vi "GEA2 Script_Parser.vi"(0 "Script path":path, 5 "Default wait time (sec)":dbl=0.25 format="%#_13g", 7 "Default continue if failed?":bool, 11 "Error In":errorcluster) -> (4 "Script Output":T1[](array[typedef]), 6 "GEA2 Script":string, 15 "Error Out":errorcluster)   [LabVIEW 2014]
uses:
  typedefs/Script Output.ctl
  typedefs/Command Type.ctl
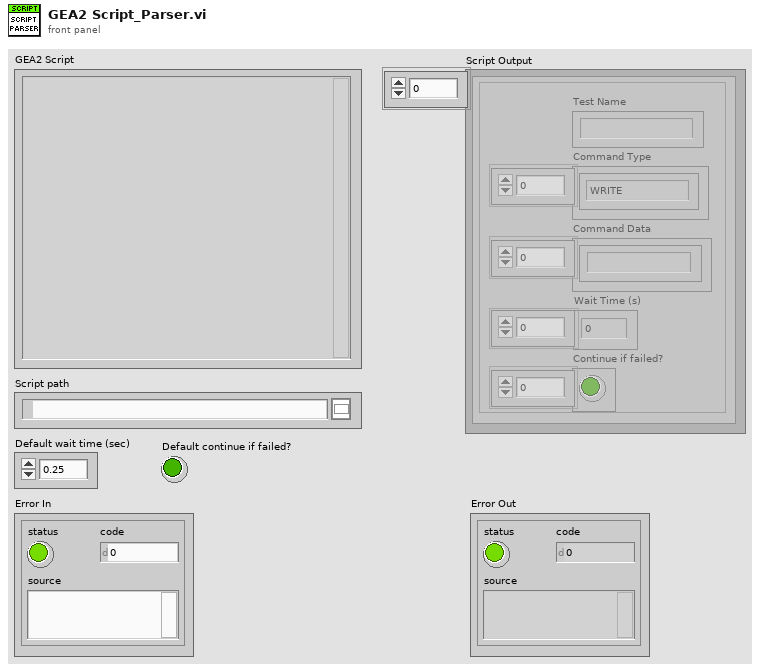
[diagram p1: front panel]
types:
  T1 = typedef "Script Output.ctl" = cluster{"Command Data":string[], "Command Type":T2[], "Test Name":string, "Wait Time (s)":dbl[], "Continue if failed?":bool[]}
  T2 = typedef "Command Type.ctl" = enum16{"WRITE", "READ", "ERDWRITE", "ERDREAD"}
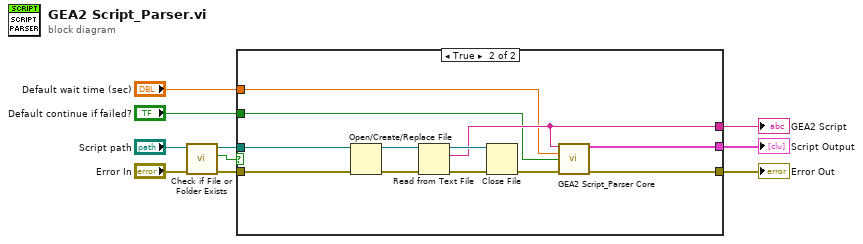
[diagram p0: block diagram]
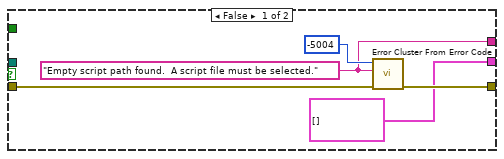
[diagram p2: hidden frame]
diagram:
  n1 = call <vilib>:"Check if File or Folder Exists.vi"("error in (no error)"="Error In", "path"="Script path") -> ("error out"=w7:errorcluster, "file or folder exists?"=w4:bool, "dup path"=w6:path)  [unwired: 7 in]
  n2 = case shown="True" w4 {
    tunnel: w7 -> [w14 w27]
    tunnel: [w15 w19] -> w10
    tunnel: "Default wait time (sec)" -> [_ w18]
    tunnel: w6 -> [_ w22]
    tunnel: [w12 w20] -> w3
    tunnel: "Default continue if failed?" -> [_ w17]
    tunnel: [T1[] [] ("Script Output") w16] -> w1
    frame False {
      w12 = "Empty script path found.  A script file must be selected." ("error message (\"\")")
      n3 = call <vilib>:"Error Cluster From Error Code.vi"("error in (no error)"=w14, "error message (\"\")"=w12, "error code (0)"=-5004) -> ("error out"=w15:errorcluster)  [unwired: 6 in]
    }
    frame True {
      n4 = Open/Create/Replace File(file path (use dialog)=w22, error in=w27) -> (refnum out=w23:refnum<file>, error out=w26:errorcluster)  [unwired: 4 in, 1 out]
      n5 = Read from Text File(file (use dialog)=w23, error in=w26) -> (refnum out=w24:refnum<file>, text=w20:string, error out=w25:errorcluster)  [unwired: 2 in, 1 out]
      n6 = Close File(refnum=w24, error in=w25) -> (error out=w21:errorcluster)  [unwired: 1 out]
      n7 = call "GEA2 Script_Parser Core.vi"("Script In"=w20, "Default wait time (s)"=w18, "Default continue if failed?"=w17, "Error In"=w21) -> ("Script Output"=w16:T1[], "Error Out"=w19:errorcluster)  [unwired: 10 in]
    }
  }
  "Error Out" <- w10
  "GEA2 Script" <- w3
  "Script Output" <- w1
